vi "RPNLogicSolverError.vi"(8 "error in":errorcluster, 9 "Variables State in":T1, 10 "HW CTRL Data":T2, 11 "Logic Parsed Expression":T3) -> (0 "error out":errorcluster, 1 "Variables State out":T1, 2 "Logic Result":bool)   [LabVIEW 2014]
doc: "Resuelve las operaciones lógicas de \"Error o Alarma\" en función del estado de las entradas digitales."
uses:
  TypeDefs/LogicParsedExpression.ctl
  TypeDefs/HW CTRL Data.ctl
  TypeDefs/HW Variables State.ctl
  SeqLoop.lvlib
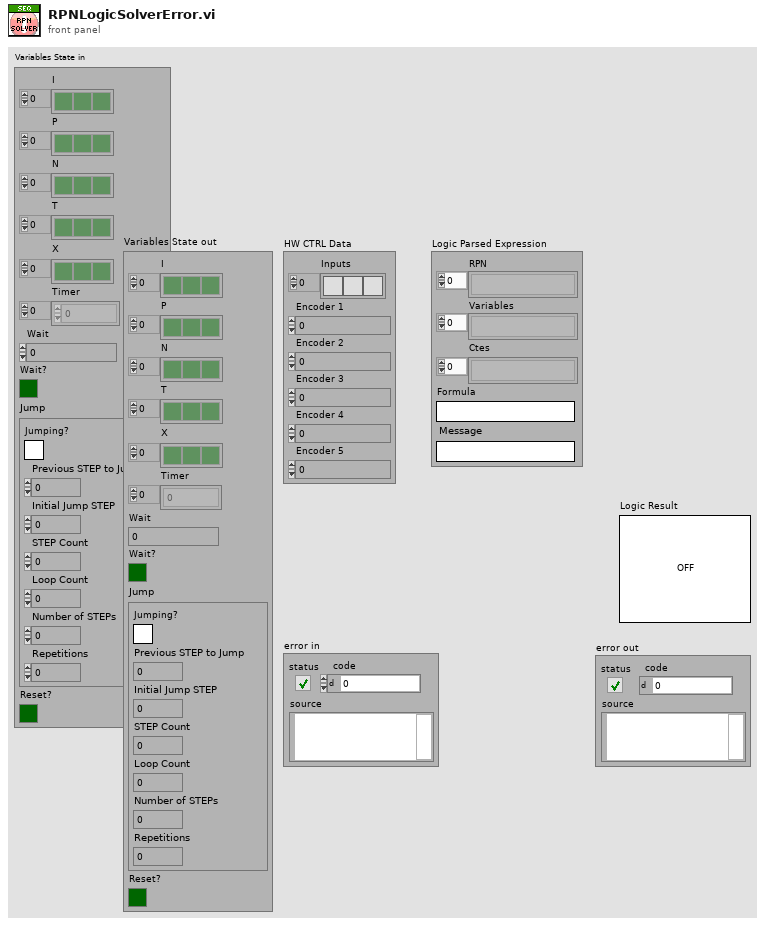
[diagram p1: front panel]
types:
  T1 = typedef "SeqLoop.lvlib/HW Variables State.ctl" = cluster{"I":bool[], "P":bool[], "N":bool[], "T":bool[], "X":bool[], "Timer":u32[], "Wait":u32, "Wait?":bool, "Jump":cluster{"Jumping?":bool, "Previous STEP to Jump":u32, "Initial Jump STEP":u32, "STEP Count":u32, "Loop Count":u32, "Number of STEPs":u32, "Repetitions":u32}, "Reset?":bool}
  T2 = typedef "SeqLoop.lvlib/HW CTRL Data.ctl" = cluster{"Inputs":bool[], "Encoder 1":sgl, "Encoder 2":sgl, "Encoder 3":sgl, "Encoder 4":sgl, "Encoder 5":sgl}
  T3 = typedef "SeqLoop.lvlib/LogicParsedExpression.ctl" = cluster{"RPN ":string[], "Variables":string[], "Ctes":string[], "Formula":string, "Message":string}
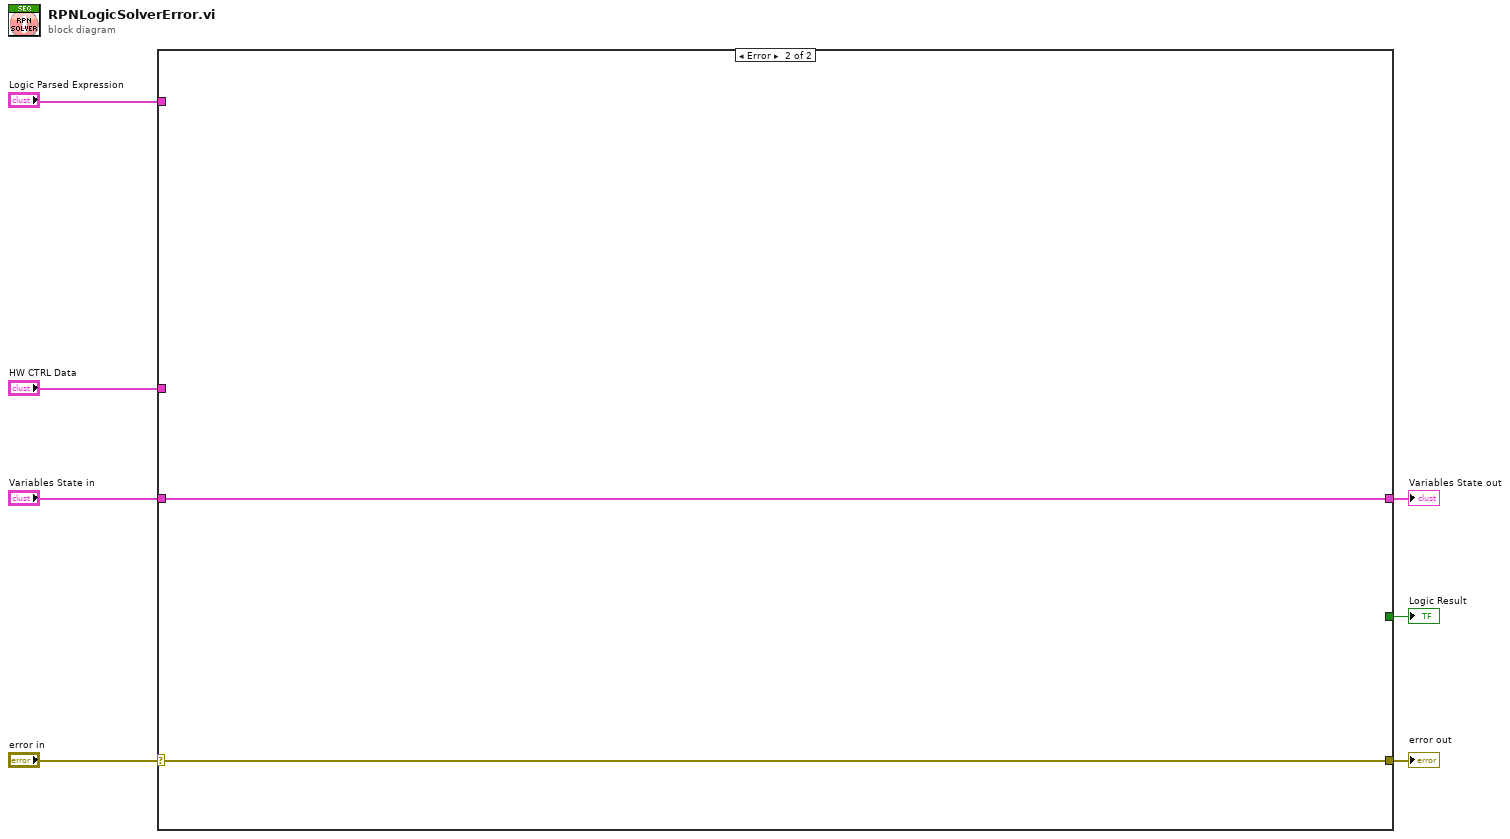
[diagram p0: block diagram]
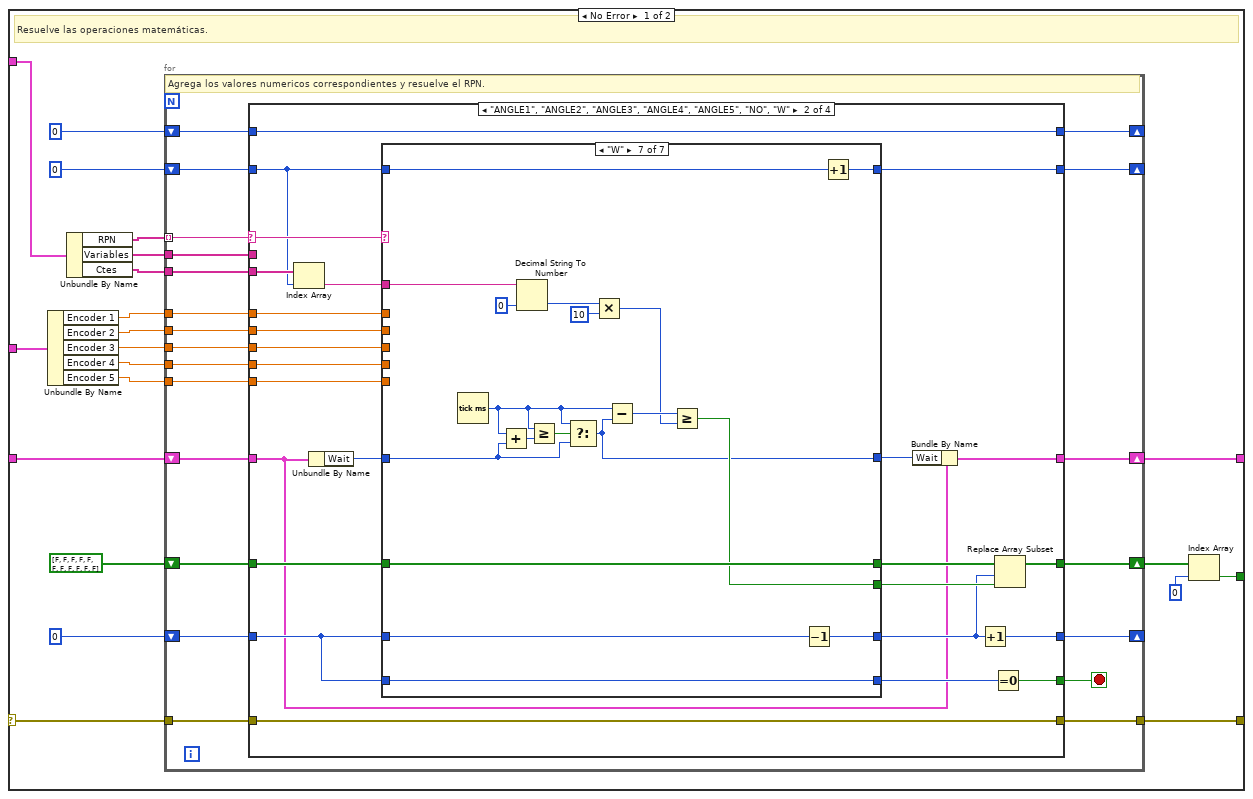
[diagram p2: hidden frame]
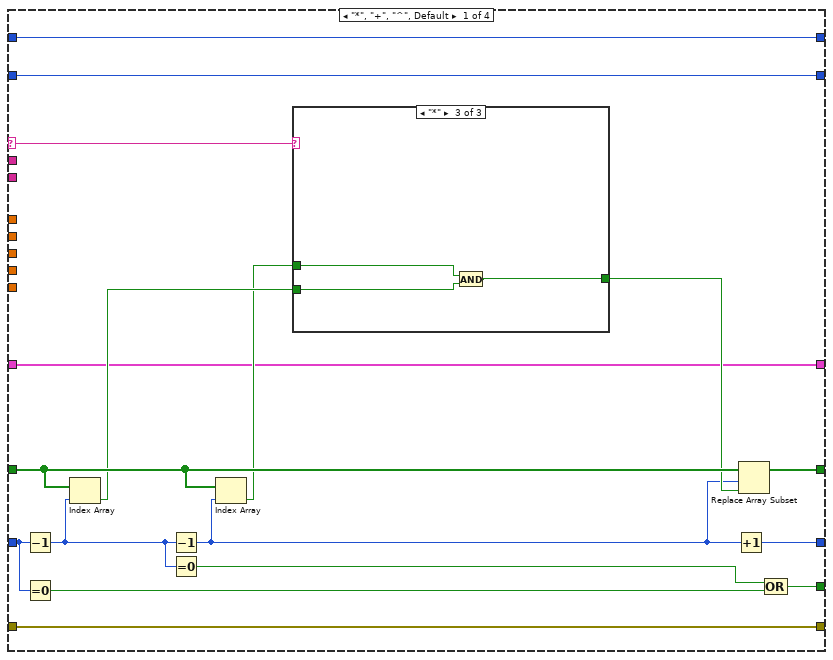
[diagram p3: hidden frame]
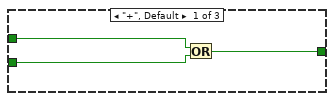
[diagram p4: hidden frame]
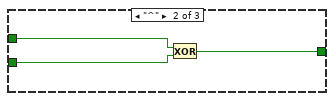
[diagram p5: hidden frame]
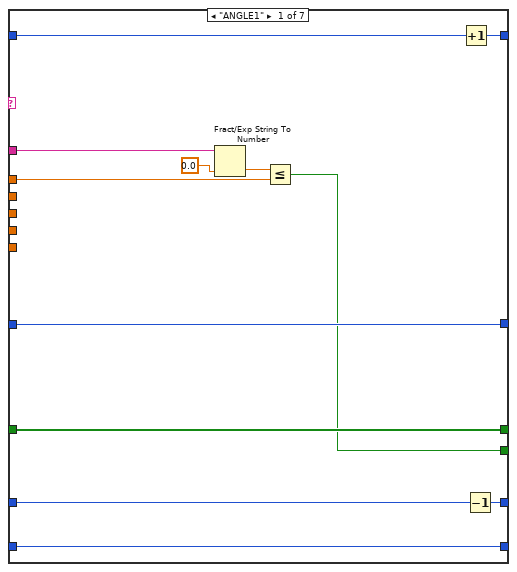
[diagram p6: hidden frame]
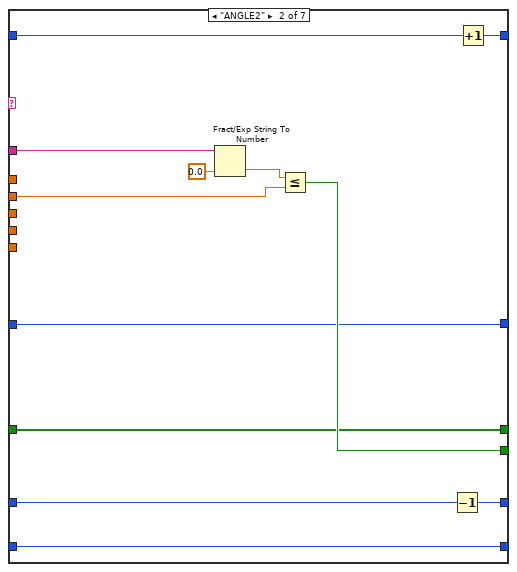
[diagram p7: hidden frame]
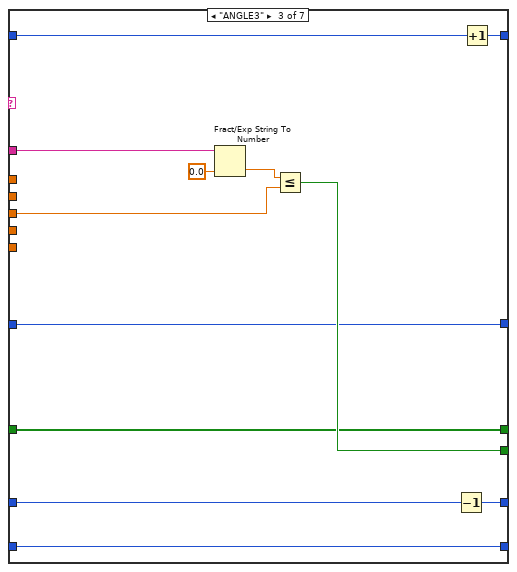
[diagram p8: hidden frame]
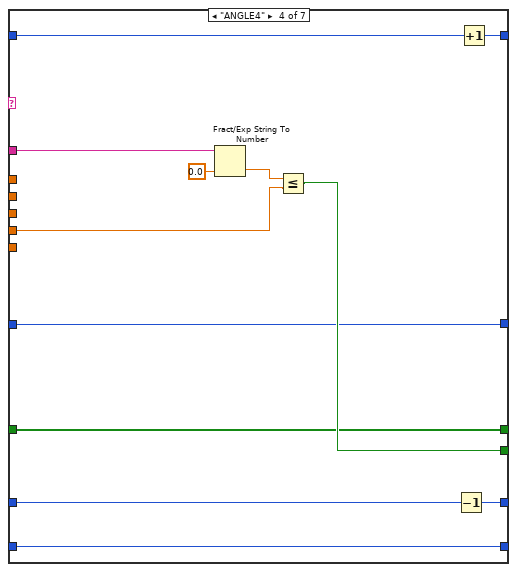
[diagram p9: hidden frame]
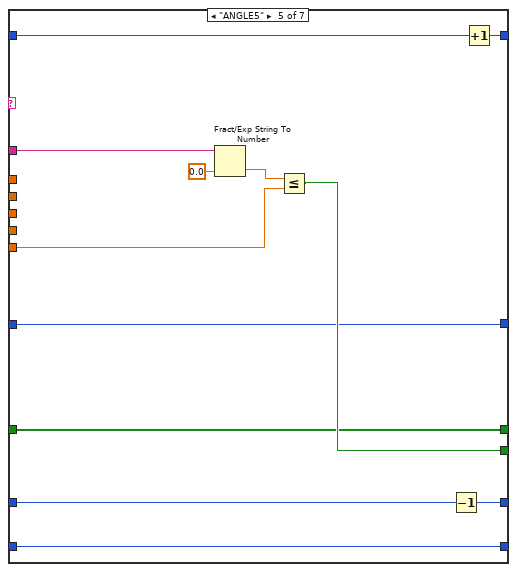
[diagram p10: hidden frame]
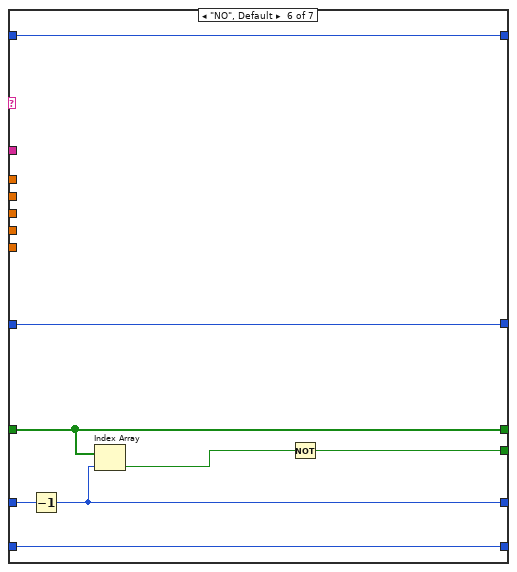
[diagram p11: hidden frame]
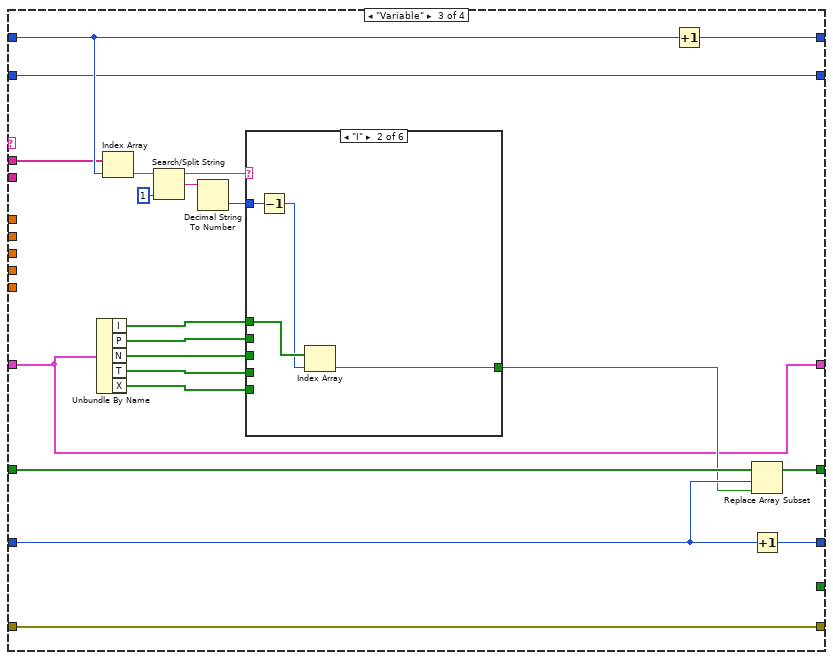
[diagram p12: hidden frame]
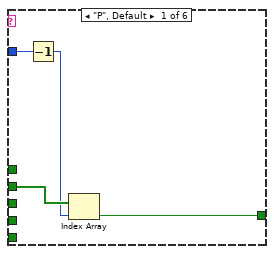
[diagram p13: hidden frame]
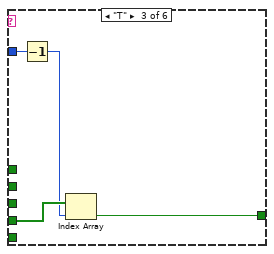
[diagram p14: hidden frame]
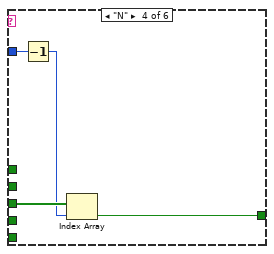
[diagram p15: hidden frame]
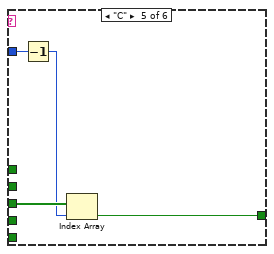
[diagram p16: hidden frame]
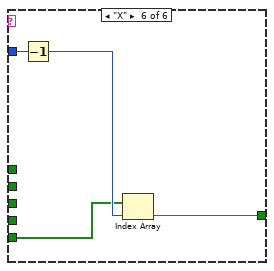
[diagram p17: hidden frame]
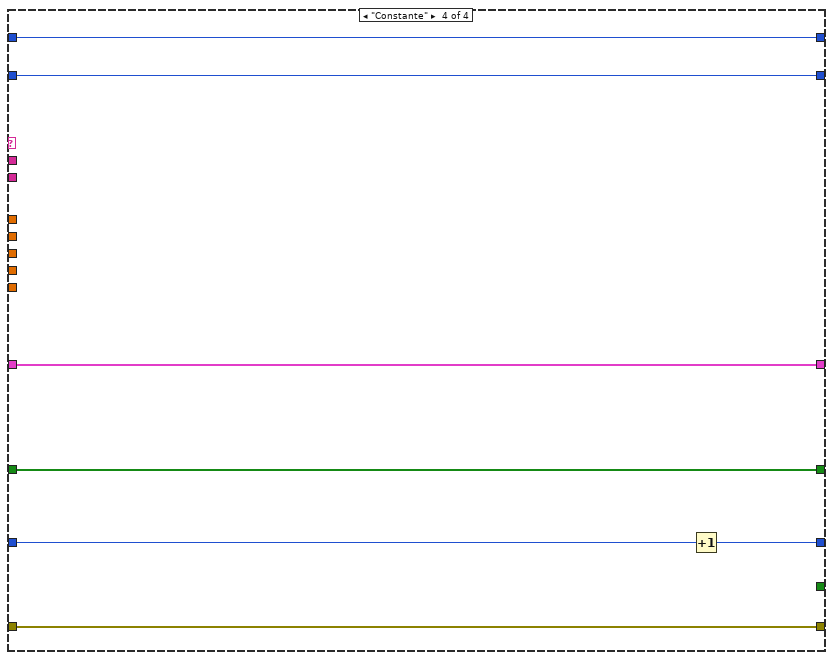
[diagram p18: hidden frame]
diagram:
  n1 = case shown="No Error" "error in" {
    selector: "error in" -> [w18 w240]
    tunnel: [w17 w240] -> w7
    tunnel: "Logic Parsed Expression" -> [w26 _]
    tunnel: [w22 _] -> w2
    tunnel: "HW CTRL Data" -> [w16 _]
    tunnel: "Variables State in" -> [w14 w239]
    tunnel: [w8 w239] -> w1
    frame No Error {
      # "Resuelve las operaciones matemáticas."
      n2 = Unbundle By Name(w16) -> ("Encoder 1"=w15:sgl, "Encoder 2"=w12:sgl, "Encoder 3"=w11:sgl, "Encoder 4"=w10:sgl, "Encoder 5"=w9:sgl)
      n3 = Unbundle By Name(w26) -> ("RPN"=w27:string[], "Variables"=w25:string[], "Ctes"=w13:string[])
      n4 = for {
        tunnel: w25 -> [w47]
        tunnel: w27 -> [w48] mode=indexing
        shift-right: [w45] -> _
        shift-left: 0 -> [w46]
        shift-right: [w44] -> _
        shift-left: 0 -> [w43]
        shift-right: [w42] -> w20
        shift-left: bool[] [FALSE, FALSE, FALSE, FALSE, FALSE, FALSE, FALSE, FALSE, FALSE, FALSE, FALSE] -> [w41]
        shift-right: [w39] -> _
        shift-left: 0 -> [w40]
        tunnel: w18 -> [w38]
        tunnel: [w37] -> w17
        tunnel: w15 -> [w36]
        tunnel: w13 -> [w34]
        tunnel: w12 -> [w33]
        tunnel: w11 -> [w32]
        tunnel: w10 -> [w31]
        tunnel: w9 -> [w30]
        shift-right: [w29] -> w8
        shift-left: w14 -> [w35]
        stop <- w49 stop-if-true
        # "Agrega los valores numericos correspondientes y resuelve el RPN."
        n5 = case shown="\"ANGLE1\", \"ANGLE2\", \"ANGLE3\", \"ANGLE4\", \"ANGLE5\", \"NO\", \"W\"" w48 {
          selector: w48 -> [w66 w93 _ _]
          tunnel: [w65 w99 _ _] -> w49
          tunnel: w47 -> [_ _ w195 _]
          tunnel: w46 -> [w64 w86 w188 w238]
          tunnel: [w64 w85 w188 w238] -> w45
          tunnel: w43 -> [w63 w100 w196 w233]
          tunnel: [w63 w100 w207 w233] -> w44
          tunnel: w41 -> [w60 w84 w205 w236]
          tunnel: [w59 w97 w204 w236] -> w42
          tunnel: w40 -> [w62 w80 w203 w235]
          tunnel: [w52 w96 w206 w234] -> w39
          tunnel: w38 -> [w51 w95 w202 w237]
          tunnel: [w51 w95 w202 w237] -> w37
          tunnel: w36 -> [_ w94 _ _]
          tunnel: w35 -> [w50 w77 w187 w232]
          tunnel: w34 -> [_ w92 _ _]
          tunnel: w33 -> [_ w90 _ _]
          tunnel: w32 -> [_ w89 _ _]
          tunnel: w31 -> [_ w88 _ _]
          tunnel: w30 -> [_ w87 _ _]
          tunnel: [w50 w76 w187 w232] -> w29
          frame "*", "+", "^", Default {
            n6 = Decrement(x=w62) -> (x-1=w61:i32)
            n7 = Equal To 0?(x=w62) -> (x = 0?=w55:bool)
            n8 = Index Array(array=w60, index=w61) -> (element=w57:bool)
            n9 = Decrement(x=w61) -> (x-1=w53:i32)
            n10 = Equal To 0?(x=w61) -> (x = 0?=w54:bool)
            n11 = Index Array(array=w60, index=w53) -> (element=w56:bool)
            n12 = case shown="\"*\"" w66 {
              tunnel: w57 -> [w67 w70 w73]
              tunnel: w56 -> [w68 w71 w74]
              tunnel: [w69 w72 w75] -> w58
              frame "+", Default {
                n13 = Or(x=w68, y=w67) -> (x .or. y?=w69:bool)
              }
              frame "^" {
                n14 = Exclusive Or(1:w70, 2:w71) -> (0:w72:bool)
              }
              frame "*" {
                n15 = And(x=w74, y=w73) -> (x .and. y?=w75:bool)
              }
            }
            n16 = Increment(x=w53) -> (x+1=w52:i32)
            n17 = Replace Array Subset(array=w60, new element=w58, index=w53) -> (w59:bool[])
            n18 = Compound Arithmetic op=OR(w54, w55) -> (w65:bool)
          }
          frame "ANGLE1", "ANGLE2", "ANGLE3", "ANGLE4", "ANGLE5", "NO", "W" {
            n19 = Index Array(array=w92, index=w86) -> (element=w91:string)
            n20 = Unbundle By Name(w77) -> ("Wait"=w79:u32)
            n21 = case shown="\"W\"" w93 {
              tunnel: [w101 w120 w132 w144 w154 w168 w170] -> w98
              tunnel: w91 -> [w112 w124 w136 w148 w160 _ w177]
              tunnel: w94 -> [w108 _ _ _ _ _ _]
              tunnel: w90 -> [_ w119 _ _ _ _ _]
              tunnel: w89 -> [_ _ w131 _ _ _ _]
              tunnel: w88 -> [_ _ _ w143 _ _ _]
              tunnel: w87 -> [_ _ _ _ w156 _ _]
              tunnel: w86 -> [w110 w122 w134 w146 w158 w167 w182]
              tunnel: [w109 w121 w133 w145 w157 w167 w181] -> w85
              tunnel: w80 -> [w105 w116 w128 w140 w152 w164 w185]
              tunnel: [w104 w115 w127 w139 w151 w163 w184] -> w82
              tunnel: w84 -> [w106 w117 w129 w141 w153 w165 w186]
              tunnel: [w106 w117 w129 w141 w153 w165 w186] -> w83
              tunnel: [w103 w114 w126 w138 w150 w162 w183] -> w81
              tunnel: w80 -> [w103 w114 w126 w138 w150 w162 w183]
              tunnel: w79 -> [w102 w113 w125 w137 w149 w161 w176]
              tunnel: [w102 w113 w125 w137 w149 w161 w169] -> w78
              frame "ANGLE1" {
                n22 = Fract/Exp String To Number(string=w112, default (0 dbl)=sgl 0.0 ("default (0 DBL)")) -> (number=w107:sgl)  [unwired: 2 in, 1 out]
                n23 = Less Or Equal?(x=w107, y=w108) -> (x <= y?=w101:bool)
                n24 = Increment(x=w110) -> (x+1=w109:i32)
                n25 = Decrement(x=w105) -> (x-1=w104:i32)
              }
              frame "ANGLE2" {
                n26 = Fract/Exp String To Number(string=w124, default (0 dbl)=sgl 0.0 ("default (0 DBL)")) -> (number=w118:sgl)  [unwired: 2 in, 1 out]
                n27 = Less Or Equal?(x=w118, y=w119) -> (x <= y?=w120:bool)
                n28 = Decrement(x=w116) -> (x-1=w115:i32)
                n29 = Increment(x=w122) -> (x+1=w121:i32)
              }
              frame "ANGLE3" {
                n30 = Fract/Exp String To Number(string=w136, default (0 dbl)=sgl 0.0 ("default (0 DBL)")) -> (number=w130:sgl)  [unwired: 2 in, 1 out]
                n31 = Less Or Equal?(x=w130, y=w131) -> (x <= y?=w132:bool)
                n32 = Decrement(x=w128) -> (x-1=w127:i32)
                n33 = Increment(x=w134) -> (x+1=w133:i32)
              }
              frame "ANGLE4" {
                n34 = Fract/Exp String To Number(string=w148, default (0 dbl)=sgl 0.0 ("default (0 DBL)")) -> (number=w142:sgl)  [unwired: 2 in, 1 out]
                n35 = Less Or Equal?(x=w142, y=w143) -> (x <= y?=w144:bool)
                n36 = Decrement(x=w140) -> (x-1=w139:i32)
                n37 = Increment(x=w146) -> (x+1=w145:i32)
              }
              frame "ANGLE5" {
                n38 = Fract/Exp String To Number(string=w160, default (0 dbl)=sgl 0.0 ("default (0 DBL)")) -> (number=w155:sgl)  [unwired: 2 in, 1 out]
                n39 = Less Or Equal?(x=w155, y=w156) -> (x <= y?=w154:bool)
                n40 = Decrement(x=w152) -> (x-1=w151:i32)
                n41 = Increment(x=w158) -> (x+1=w157:i32)
              }
              frame "NO", Default {
                n42 = Decrement(x=w164) -> (x-1=w163:i32)
                n43 = Index Array(array=w165, index=w163) -> (element=w166:bool)
                n44 = Not(x=w166) -> (.not. x?=w168:bool)
              }
              frame "W" {
                n45 = Tick Count (ms)() -> (millisecond timer value=w178:u32)
                n46 = Add(x=w178, y=w176) -> (x+y=w179:u32)
                n47 = Decimal String To Number(string=w177, default (0L)=u32 0 ("default (0 I32)")) -> (number=w172:u32)  [unwired: 1 in, 1 out]
                n48 = Greater Or Equal?(x=w178, y=w179) -> (x >= y?=w180:bool)
                n49 = Select(t=w178, s=w180, f=w176) -> (s? t:f=w169:u32)
                n50 = Multiply(x=w172, y=u32 10) -> (x*y=w171:u32)
                n51 = Subtract(x=w178, y=w169) -> (x-y=w174:u32)
                n52 = Greater Or Equal?(x=w174, y=w171) -> (x >= y?=w170:bool)
                n53 = Decrement(x=w185) -> (x-1=w184:i32)
                n54 = Increment(x=w182) -> (x+1=w181:i32)
              }
            }
            n55 = Bundle By Name(cluster=w77, "Wait"=w78) -> (w76:T1)
            n56 = Increment(x=w82) -> (x+1=w96:i32)
            n57 = Equal To 0?(x=w81) -> (x = 0?=w99:bool)
            n58 = Replace Array Subset(array=w83, new element=w98, index=w82) -> (w97:bool[])
          }
          frame "Variable" {
            n59 = Unbundle By Name(w187) -> ("I"=w193:bool[], "P"=w190:bool[], "N"=w192:bool[], "T"=w191:bool[], "X"=w189:bool[])
            n60 = Index Array(array=w195, index=w196) -> (element=w194:string)
            n61 = Search/Split String(string=w194, offset (0)=1 ("length (rest)")) -> (substring before match=w200:string, match + rest of string=w199:string)  [unwired: 1 in, 1 out]
            n62 = Decimal String To Number(string=w199) -> (number=w198:i32)  [unwired: 2 in, 1 out]
            n63 = case shown="\"I\"" w200 {
              tunnel: w198 -> [w209 w213 w217 w221 w225 w230]
              tunnel: [w211 w215 w219 w223 w227 w231] -> w197
              tunnel: w193 -> [_ w214 _ _ _ _]
              tunnel: w190 -> [w210 _ _ _ _ _]
              tunnel: w192 -> [_ _ _ w222 w226 _]
              tunnel: w191 -> [_ _ w218 _ _ _]
              tunnel: w189 -> [_ _ _ _ _ w228]
              frame "P", Default {
                n64 = Decrement(x=w209) -> (x-1=w208:i32)
                n65 = Index Array(array=w210, index=w208) -> (element=w211:bool)
              }
              frame "I" {
                n66 = Decrement(x=w213) -> (x-1=w212:i32)
                n67 = Index Array(array=w214, index=w212) -> (element=w215:bool)
              }
              frame "T" {
                n68 = Decrement(x=w217) -> (x-1=w216:i32)
                n69 = Index Array(array=w218, index=w216) -> (element=w219:bool)
              }
              frame "N" {
                n70 = Decrement(x=w221) -> (x-1=w220:i32)
                n71 = Index Array(array=w222, index=w220) -> (element=w223:bool)
              }
              frame "C" {
                n72 = Decrement(x=w225) -> (x-1=w224:i32)
                n73 = Index Array(array=w226, index=w224) -> (element=w227:bool)
              }
              frame "X" {
                n74 = Decrement(x=w230) -> (x-1=w229:i32)
                n75 = Index Array(array=w228, index=w229) -> (element=w231:bool)
              }
            }
            n76 = Increment(x=w196) -> (x+1=w207:i32)
            n77 = Replace Array Subset(array=w205, new element=w197, index=w203) -> (w204:bool[])
            n78 = Increment(x=w203) -> (x+1=w206:i32)
          }
          frame "Constante" {
            n79 = Increment(x=w235) -> (x+1=w234:i32)
          }
        }
      }
      n80 = Index Array(array=w20, index=0) -> (element=w22:bool)
    }
    frame Error {
    }
  }
  "error out" <- w7
  "Logic Result" <- w2
  "Variables State out" <- w1
